vi "Criar Evento de Usuário.vi"(8 "error in (no error)":errorcluster) -> (0 "error out":errorcluster, 3 "Event Registration Refnum":refnum<event-registration>)   [LabVIEW 2020]
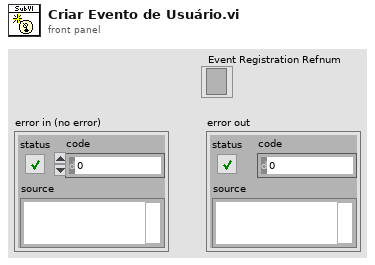
[diagram p1: front panel]
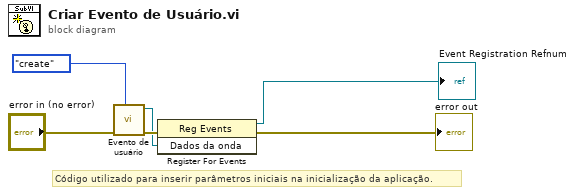
[diagram p0: block diagram]
diagram:
  # "Código utilizado para inserir parâmetros iniciais na inicialização da aplicação."
  n1 = call "Evento de usuário.vi"("Enum"=enum16{"create", "fire", "destroy"}."create", "error in (no error)"="error in (no error)") -> ("error out"=w4:errorcluster, "Dados da onda"=w2:refnum<user-event>)  [unwired: 8 in]
  n2 = register-events(error in=w4, w2) -> (reference out=→"Event Registration Refnum":refnum<event-registration>, error out=→"error out":errorcluster)  [unwired: 1 in]
